vi "test_Create Global MetaData Channel_after adding a IA CD.vi"(8 "error in (no error)":errorcluster, 11 "TestCase in":refnum<class "Instrument Addon Scripting API Channels Unit Tests.lvclass">) -> (0 "error out":errorcluster, 3 "TestCase out":refnum<class "Instrument Addon Scripting API Channels Unit Tests.lvclass">)   [LabVIEW 2019, in "Instrument Addon Scripting API Channels Unit Tests.lvclass"]
uses:
  Instrument Addon Scripting API Channels Unit Tests.lvclass
  <vilib>/addons/_JKI Toolkits/VI Tester/TestCase.llb/TestCase.lvclass
  <vilib>/NI VeriStand/Custom Device Tools/Custom Device Utility Library/Custom Device Utility Library.lvlib
  Addon/Addon Shared/SubVIs/Constants.vi
  Addon/Addon Shared/Instrument Addon Shared.lvlib
  Addon/Addon Shared/Types/FG Control.ctl
  APIs/Scripting API/Instrument Addon Scripting API.lvlib
  APIs/Scripting API/TypeDefs/Array Element.ctl
  APIs/Scripting API/TypeDefs/Array Enumerated List Settings.ctl
  Includes/Protocols.lvlibp/TCP/TCP Settings.ctl
  Includes/Protocols.lvlibp/TCP/TCP.lvclass
  <vilib>/NI VeriStand/Custom Device Tools/Custom Device Utility Library/NI VeriStand - Search for Item by Name.vi
  APIs/Scripting API/Channels/Create Global MetaData Channel - Array - Enumerated List.vi
  <vilib>/NI VeriStand/Custom Device Tools/Custom Device Utility Library/NI VeriStand - Search for Item by GUID.vi
  APIs/Scripting API/Custom Device/TCP Factory.vi
  C:/Program Files (x86)/National Instruments/LabVIEW 2019/vi.lib/addons/_JKI Toolkits/VI Tester/TestCase.llb/TestCase.lvclass
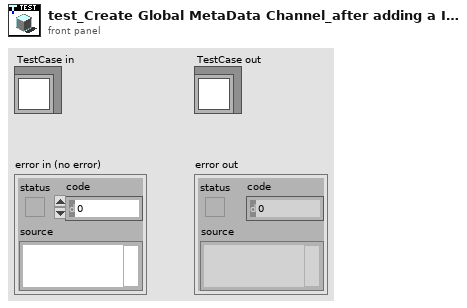
[diagram p1: front panel]
types:
  T1 = typedef "Protocols.lvlibp/TCP.lvclass/TCP Settings.ctl" = cluster{"IP Address":string, "Port":u16}
  T2 = typedef "Instrument Addon Shared.lvlib/FG Control.ctl" = enum16{"Get", "Set"}
  T3 = typedef "Instrument Addon Scripting API.lvlib/Array Enumerated List Settings.ctl" = cluster{"Elements":T4[], "Enumerated List":string[], "Delimiter":string}
  T4 = typedef "Instrument Addon Scripting API.lvlib/Array Element.ctl" = cluster{"Name":string, "Default Value":dbl, "Units":string}
  T5 = typedef "Custom Device API.lvlib/Custom Device Item Ref.ctl" = u64
  T6 = typedef "Instrument Addon Shared.lvlib/MetaData Parameters.ctl" = cluster{"Data Type":T7, "Channel Type":T8, "List":string[], "Format String":string, "Type":T9, "Delimiter":string, "Endian":T10}
  T7 = typedef "Instrument Addon Shared.lvlib/Protocol Data Type.ctl" = enum16{"Single Channel", "Array"}
  T8 = typedef "Instrument Addon Shared.lvlib/Metadata Channel Type.ctl" = enum16{"Enumerated List", "Format", "Type Cast"}
  T9 = typedef "Instrument Addon Shared.lvlib/Type Cast Type.ctl" = enum16{"DBL", "SGL", "U64", "U32", "U16", "U8", "I64", "I32", "I16", "I8"}
  T10 = typedef "Instrument Addon Shared.lvlib/Endian.ctl" = enum16{"Native", "Little", "Big"}
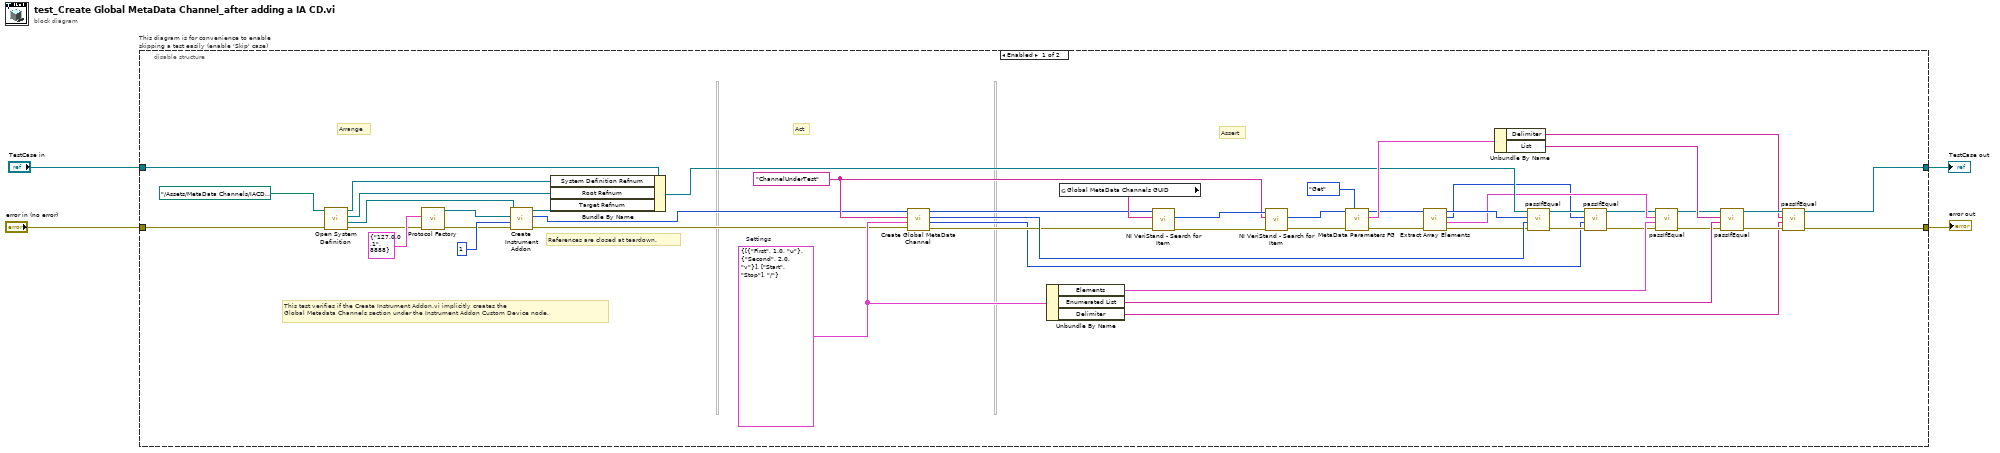
[diagram p0: block diagram]
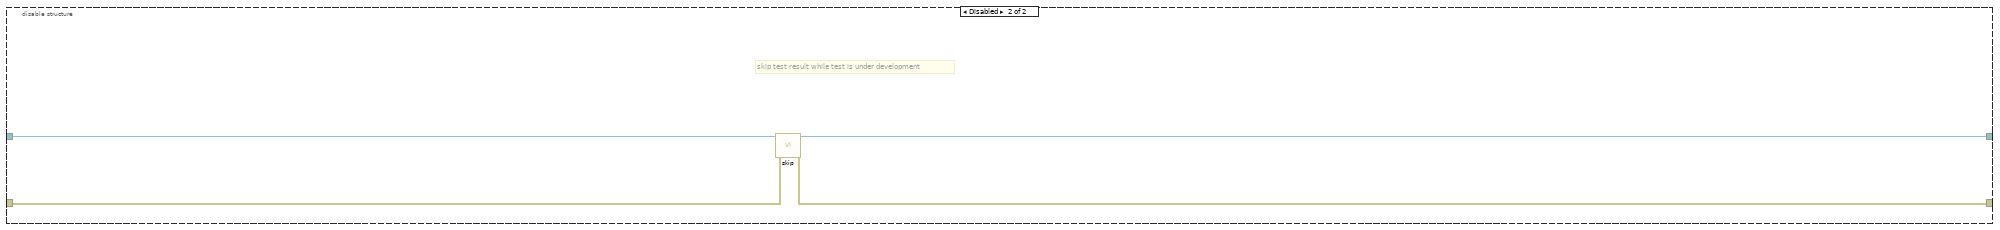
[diagram p2: hidden frame]
diagram:
  n1 = disable-structure "This diagram is for convenience to enable skipping a test easily (enable 'Skip' case)" shown="Enabled" {
    disable-tunnel: "TestCase in" -> [w38 w57]
    disable-tunnel: [w30 w55] -> w1
    disable-tunnel: [w29 w56] -> w3
    disable-tunnel: "error in (no error)" -> [w53 w54]
    frame Enabled {
      w33 = T3 {"Elements"=[{"Name"="First", "Default Value"=1.0, "Units"="u"}, {"Name"="Second", "Default Value"=2.0, "Units"="v"}], "Enumerated List"=["Start", "Stop"], "Delimiter"="/"}  # Settings
      w37 = "ChannelUnderTest" ("Name")
      # "This test verifies if the Create Instrument Addon.vi implicitly creates the \nGlobal Metadata Channels section under the Instrument Addon Custom Device node."
      # "References are closed at teardown."
      # "Assert"
      # "Act"
      # "Arrange"
      n2 = call "Open System Definition.vi"("error in (no error)"=w53, "System Definition File"=path "../Assets/MetaData Channels/IACD channels_EmptySysdef.nivssdf") -> ("error out"=w6:errorcluster, "Target Refnum"=w13:refnum<k24>, "Root Refnum"=w41:refnum<k24>, "System Definition Refnum"=w40:refnum<k24>)  [unwired: 6 in]
      n3 = call-poly "Protocol Factory.vi"("error in (no error)"=w6, "settings"=T1 {"IP Address"="127.0.0.1", "Port"=8888} ("TCP settings")) -> ("error out"=w5:errorcluster, "protocol out"=w7:refnum<class "Protocol Parent.lvclass">)  [unwired: 8 in]
      n4 = call "Create Instrument Addon.vi"("error in (no error)"=w5, "PCL decimation"=u16 1, "protocol in"=w7, "target in"=w13) -> ("error out"=w10:errorcluster, "instrument addon refnum"=w9:T5, "target out"=w11:refnum<k24>)  [unwired: 5 in]
      n5 = Bundle By Name(cluster=w38, "System Definition Refnum"=w40, "Root Refnum"=w41, "Target Refnum"=w11) -> (w39:refnum<class "Instrument Addon Scripting API Channels Unit Tests.lvclass">)
      n6 = call-poly "Create Global MetaData Channel.vi"("error in (no error)"=w10, "settings"=w33, "channel name"=w37, "instrument addon refnum in"=w9) -> ("error out"=w34:errorcluster, "channel refnums"=w15:T5[], "array refnum"=w35:T5, "instrument addon refnum out"=w36:T5)  [unwired: 4 in]
      n7 = Unbundle By Name(w33) -> ("Elements"=w26:T4[], "Enumerated List"=w42:string[], "Delimiter"=w32:string)
      n8 = global read "Constants.vi" "Global MetaData Channels GUID"() -> (w52:string)
      n9 = call-poly <vilib>:"NI VeriStand - Search for Item.vi"("error in"=w34, "Item GUID"=w52, "Section Ref in"=w36) -> ("error out"=w50:errorcluster, "Item Ref"=w51:T5)  [unwired: 5 in, 2 out]
      n10 = call-poly <vilib>:"NI VeriStand - Search for Item.vi"("error in"=w50, "Item Name"=w37, "Section Ref in"=w51) -> ("error out"=w49:errorcluster, "Item Ref"=w48:T5)  [unwired: 5 in, 2 out]
      n11 = call "MetaData Parameters FG.vi"("Action"=FG_Control."Get", "error in (no error)"=w49, "Item Ref in"=w48) -> ("error out"=w25:errorcluster, "MetaData Parameters"=w46:T6, "Item Ref out"=w24:T5)  [unwired: 6 in]
      n12 = call "Extract Array Elements.vi"("error in (no error)"=w25, "array reference in"=w24) -> ("error out"=w23:errorcluster, "elements"=w21:T4[], "channel refnums"=w16:T5[], "array reference out"=w22:T5)  [unwired: 6 in]
      n13 = Unbundle By Name(w46) -> ("Delimiter"=w31:string, "List"=w43:string[])
      n14 = call-dynamic "passIfEqual.vi"("error in (no error)"=w23, "y"=w35, "x"=w22, "TestCase in"=w39) -> ("error out"=w20:errorcluster, "TestCase out"=w18:refnum<class "Instrument Addon Scripting API Channels Unit Tests.lvclass">)  [unwired: 6 in]
      n15 = call-dynamic "passIfEqual.vi"("error in (no error)"=w20, "y"=w15, "x"=w16, "TestCase in"=w18) -> ("error out"=w19:errorcluster, "TestCase out"=w17:refnum<class "Instrument Addon Scripting API Channels Unit Tests.lvclass">)  [unwired: 6 in]
      n16 = call-dynamic "passIfEqual.vi"("error in (no error)"=w19, "y"=w26, "x"=w21, "TestCase in"=w17) -> ("error out"=w27:errorcluster, "TestCase out"=w28:refnum<class "Instrument Addon Scripting API Channels Unit Tests.lvclass">)  [unwired: 6 in]
      n17 = call-dynamic "passIfEqual.vi"("error in (no error)"=w27, "y"=w42, "x"=w43, "TestCase in"=w28) -> ("error out"=w45:errorcluster, "TestCase out"=w44:refnum<class "Instrument Addon Scripting API Channels Unit Tests.lvclass">)  [unwired: 6 in]
      n18 = call-dynamic "passIfEqual.vi"("error in (no error)"=w45, "y"=w32, "x"=w31, "TestCase in"=w44) -> ("error out"=w29:errorcluster, "TestCase out"=w30:refnum<class "Instrument Addon Scripting API Channels Unit Tests.lvclass">)  [unwired: 6 in]
    }
    frame Disabled {
      # "skip test result while test is under development"
      n19 = call <vilib>:"skip.vi"("error in (no error)"=w54, "TestCase in"=w57) -> ("error out"=w56:errorcluster, "TestCase out"=w55:refnum<class "Instrument Addon Scripting API Channels Unit Tests.lvclass">)  [unwired: 8 in]
    }
  }
  "error out" <- w3
  "TestCase out" <- w1
